vi "Optimal Frequency Bands Search.vi"() -> ()   [LabVIEW 2016]
uses:
  particle_swarm_opt/PSO_tParameters.ctl
  GA_core/GA_tParameters.ctl
  4. Accuracy Assessment for EEG Classification/_vlib/CU_ClassifierTypes.ctl
  <vilib>/Math Plots/2D Math Plots/2D Error Bar/2D Error Bar XCtrl/2D Error Bar.xctl
  4. Accuracy Assessment for EEG Classification/_vlib/CU_ClassifierQualityMeasure.ctl
  _vlib/OFBS_AlgorithmTypes.ctl
  _vlib/OFBS_metaParameters.ctl
  <vilib>/Math Plots/2D Math Plots/2D Error Bar/2D Error Bar Datatype/Public/Plot Helper (Fixed).vi
  4. Accuracy Assessment for EEG Classification/Classifier.lvlib
  <vilib>/Math Plots/2D Math Plots/2D Error Bar/2D Error Bar Datatype/2D Error Bar Datatype.lvclass
  <vilib>/Analysis/NI_AALBase.lvlib
  Optimal Frequency Bands Search.lvlib
  GA_core/GeneticAlgorithm.lvlib
  particle_swarm_opt/ParticleSwarm.lvlib
panel:
  in  "Stop Button":bool
  in  "Tab Control":T1(tab)
  in  "Algorithm Types":T2(tab)
  in  "GA parameters":T3={"Population size"=100, "Generations no."=20, "Significant digits"=5, "Crossover probabality"=0.85, "Mutation mode"=enum."one-point, fixed rate", "Use Gray code?"=TRUE, "Mutation rate"=0.05, "Min mutation rate"=0.0005, "Max mutation rate"=0.25, "Reproduction plan"=enum."Steady-state-replace-worst", "Elitism"=FALSE, "Fmax"=30} {"Max mutation rate" min=0.0 max=1.0; "Min mutation rate" min=0.0 max=1.0; "Mutation rate" min=0.0 max=1.0; "Crossover probabality" min=0.0 max=1.0; "Significant digits" min=1; "Generations no." min=1; "Population size" min=1}
  in  "PSO parameters":T4={"Swarm size"=100, "Generations no."=20, "Cognitive coeff a1"=2.05, "Social coeff a2"=2.05, "Min inertia weight"=0.4, "Max inertia weight "=0.9, "Fmax"=50} {"Generations no." min=1; "Swarm size" min=1}
  in  "Optimization Algorithm":T5 caption="Алгоритм поиска"
  in  "Number of Channels":i32=14 caption="Число каналов в записи ЭЭГ" min=1 max=128 step=1
  in  "ClassifierQualityMeasure":T6 caption="Критерий оценки точности классификации"
  in  "Use equal number of trials?":bool caption="Включить балансировку классов?"
  in  "Classifier Metaparameter":dbl=5.0 caption="Свободный параметр классификатора" min=0.0 max=100.0 step=0.1 format="%#_2g"
  in  "Iterations Num":i32=5
  in  "Training data paths":path[](array[path]) caption="Пути к файлам с обучающими данными"
  in  "Test data paths":path[](array[path]) caption="Пути к файлам с тестовыми данными"
  in  "True labels for Test data":path[](array[path]) caption="Пути к файлам с метками классов (для тестовых данных)"
  in  "ClassifierType":T7=enum."k NN Classifier" caption="Тип классификатора"
  in  "Start GA":bool
  out "Dataset Num":i32
  out "Total Progress":i32(slide) scale=0.0..25.0
  out "Solution":i32(listbox) caption="Оценки точности для решений, полученные после запусков поиска"
  out "Fitness Chart":cluster{i32[], dbl[]}[](graph) caption="Графики точности классификации"
  out "Accuracies":i32(listbox) caption="Оценки точности классификации на итерациях алгоритма поиска"
  out "Iteration":i32
  out "Results":string caption="Протокол выполнения программы"
  out "Accuracies out":dbl[][](array[numeric]) caption="Результаты"
  out "2D Error Bar":refnum<class "2D Plot Datatype.lvclass">[](xcontrol) caption="График средней точности классификации"
  # "This VI is a part of BCI Design library, http://www.ru-bci.org \nCopyright © 2020, Sotnikov Peter, All rights reserved. License: CC BY-NC 4.0"
  # "Параметры алгоритмов поиска"
  # "Число запусков ГА для каждого набора данных"
  # "Значение nu для SVM-классификатора (0,0 .. 1,0)\nЧисло соседей k для kNN-классификатора (1 .. 100)\nЧисло нейронов N скрытого слоя для многослойного персептрона (1 .. 100)"
  # "Размер популяции"
  # "Число поколений"
  # "Разрядность генома"
  # "Вероятность скрещивания"
  # "Тип мутаций"
  # "Использовать код Грея\nдля кодирования генома?"
  # "Вероятность мутации"
  # "Тип смены поколений"
  # "Fmax - верхняя граница частотного диапазона, \nFmin = 0"
  # "Размер роя"
  # "Число поколений"
  # "Коэффициент собственного лучшего значения"
  # "Коэффициент группового лучшего значения"
  # "Минимальное значение коэффициента инерции"
  # "Максимальное значение коэффициента инерции"
  # "Fmax - верхняя граница частотного диапазона, \nFmin = 0"
  # "Общее выполнение"
  # "Набор данных №"
  # "Запуск ГА №"
  # "Среднее \nпо наборам"
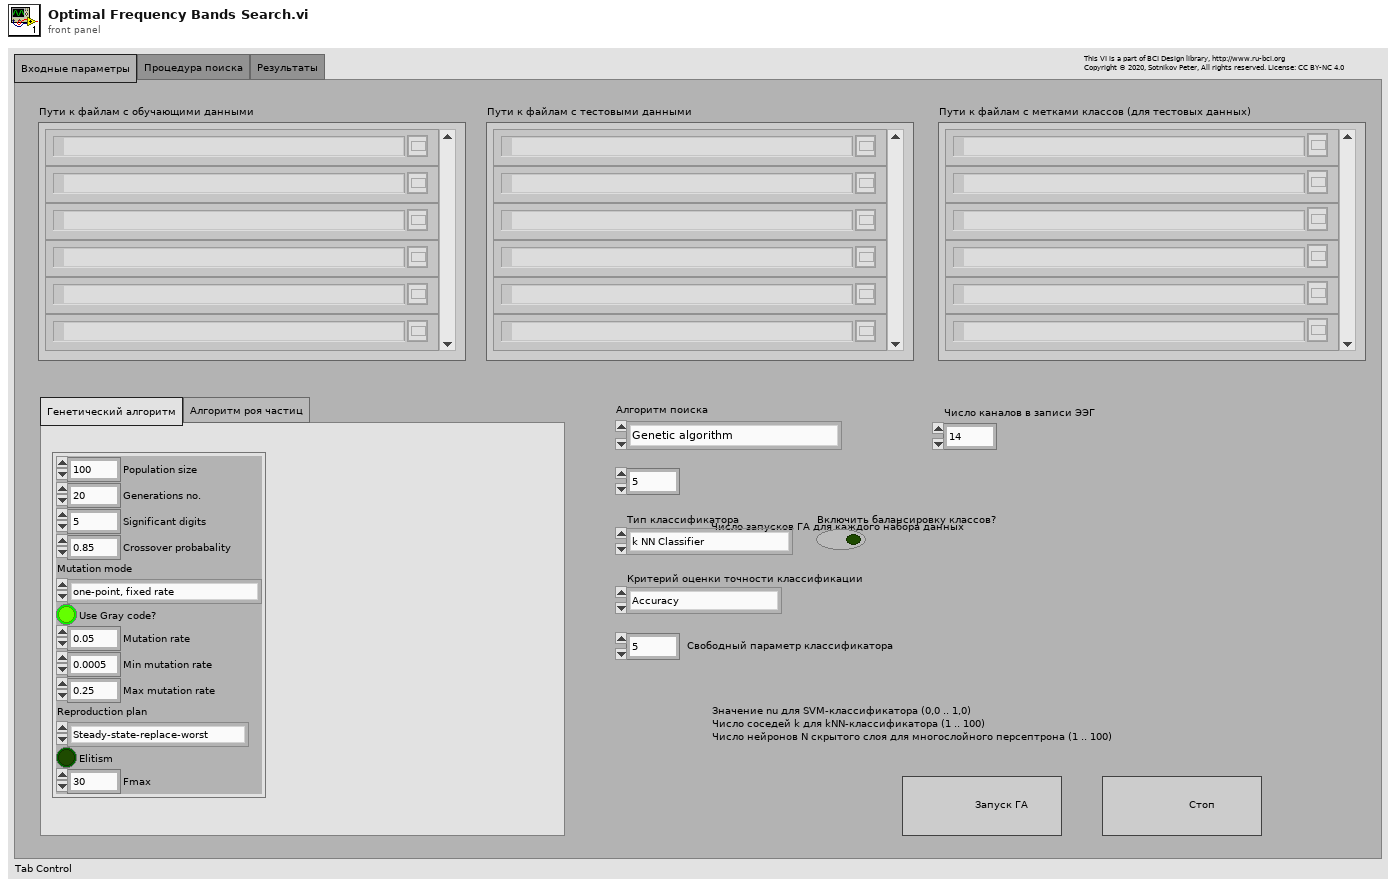
[diagram p1: front panel]
types:
  T1 = enum32{"Входные параметры", "Процедура поиска", "Результаты"}
  T2 = enum32{"Генетический алгоритм", "Алгоритм роя частиц"}
  T3 = typedef "Optimal Frequency Bands Search.lvlib/GeneticAlgorithm.lvlib/GA_tParameters.ctl" = cluster{"Population size":i32, "Generations no.":i32, "Significant digits":i32, "Crossover probabality":dbl, "Mutation mode":enum16{"one-point, fixed rate", "one-point, fitness-adjustable rate", "one-point, distance-adjustable rate"}, "Use Gray code?":bool, "Mutation rate":dbl, "Min mutation rate":dbl, "Max mutation rate":dbl, "Reproduction plan":enum16{"Full generational replacement", "Steady-state-replace-random", "Steady-state-replace-worst"}, "Elitism":bool, "Fmax":i32}
  T4 = typedef "Optimal Frequency Bands Search.lvlib/ParticleSwarm.lvlib/PSO_tParameters.ctl" = cluster{"Swarm size":i32, "Generations no.":i32, "Cognitive coeff a1":dbl, "Social coeff a2":dbl, "Min inertia weight":dbl, "Max inertia weight ":dbl, "Fmax":i32}
  T5 = typedef "Optimal Frequency Bands Search.lvlib/OFBS_AlgorithmTypes.ctl" = enum16{"Genetic algorithm", "Particle swarm optimization"}
  T6 = typedef "Classifier.lvlib/CU_ClassifierQualityMeasure.ctl" = enum16{"Accuracy", "Cohen's kappa"}
  T7 = typedef "Classifier.lvlib/CU_ClassifierTypes.ctl" = enum16{"Multilayer perceptron", "k NN Classifier", "SVM Committee", "Mahalanobis distance", "SVM Classifier"}
  T8 = typedef "Optimal Frequency Bands Search.lvlib/OFBS_metaParameters.ctl" = cluster{"Training Data Path":path, "Test Data Path":path, "True Labels for Test Trials":path, "Optimization Algorithm":T5, "ClassifierType":T7, "GA Parameters":T3, "PSO Parameters":T4, "Number of Channels":i32, "Use equal number of trials?":bool, "Classifier Metaparameter":dbl, "ClassifierQualityMeasure":T6}
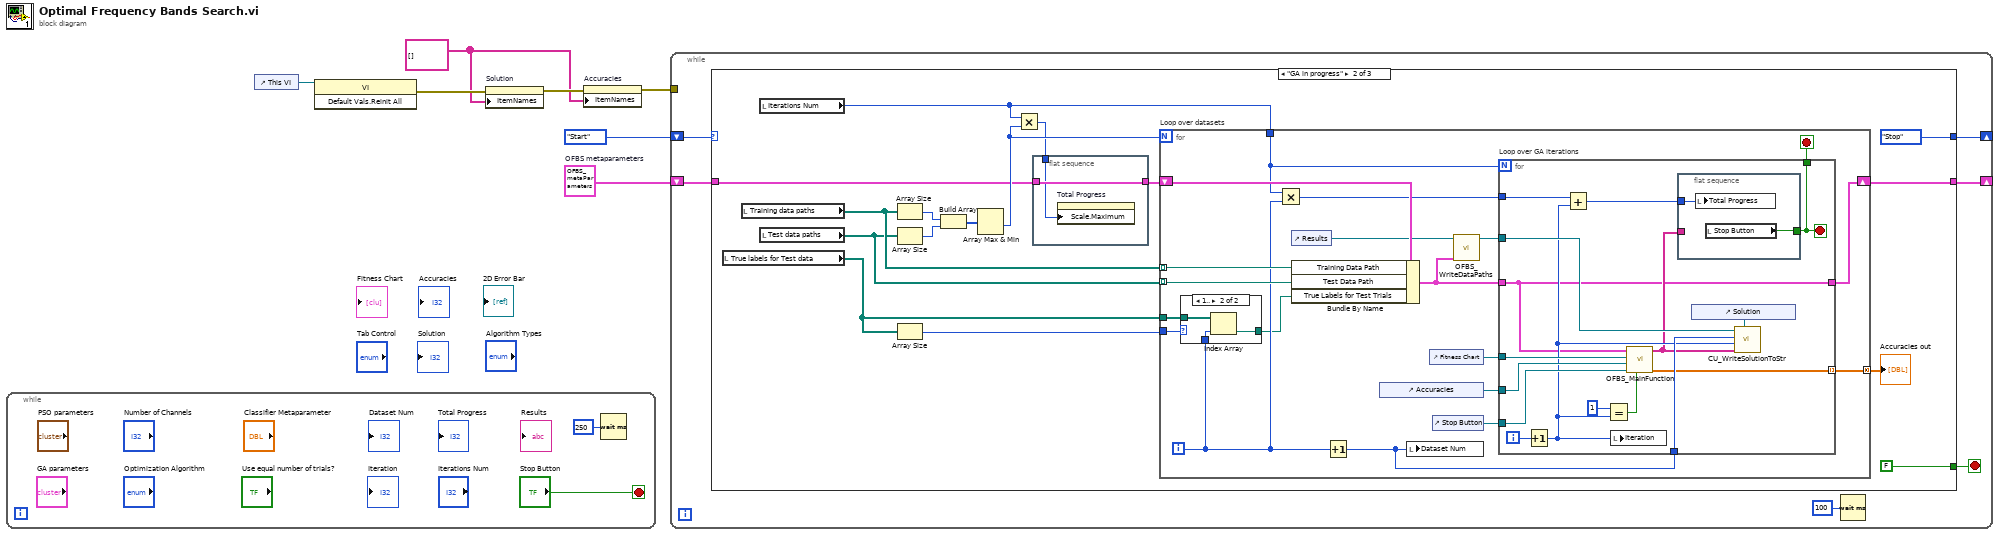
[diagram p0: block diagram]
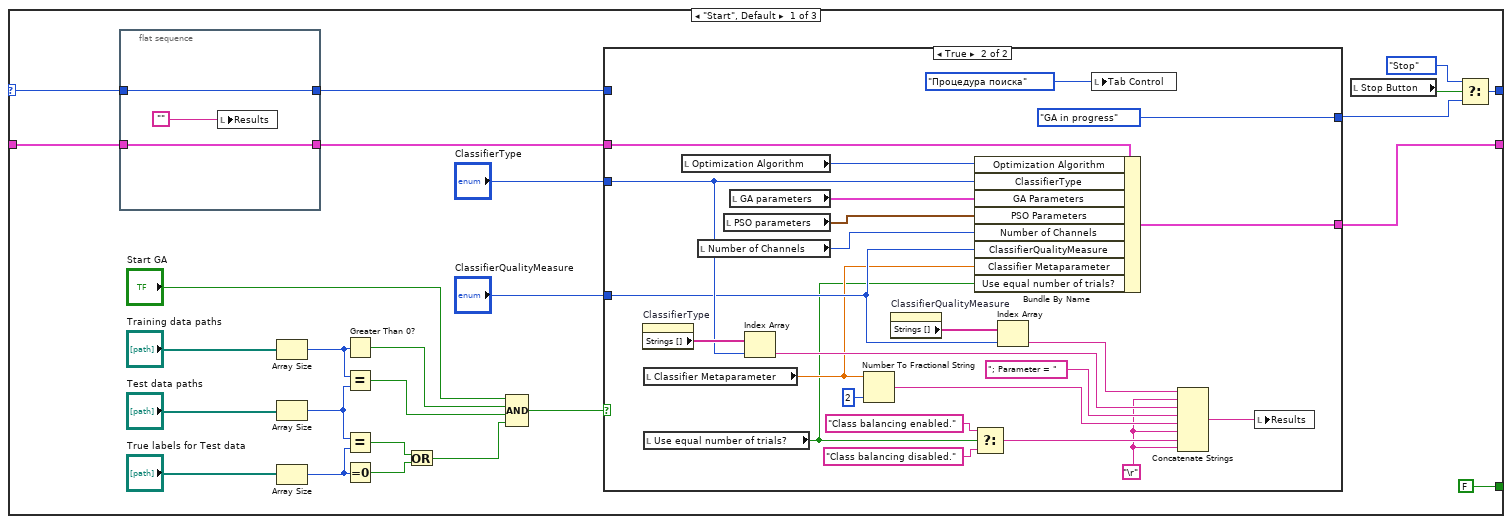
[diagram p2: hidden frame]
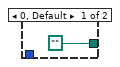
[diagram p4: hidden frame]
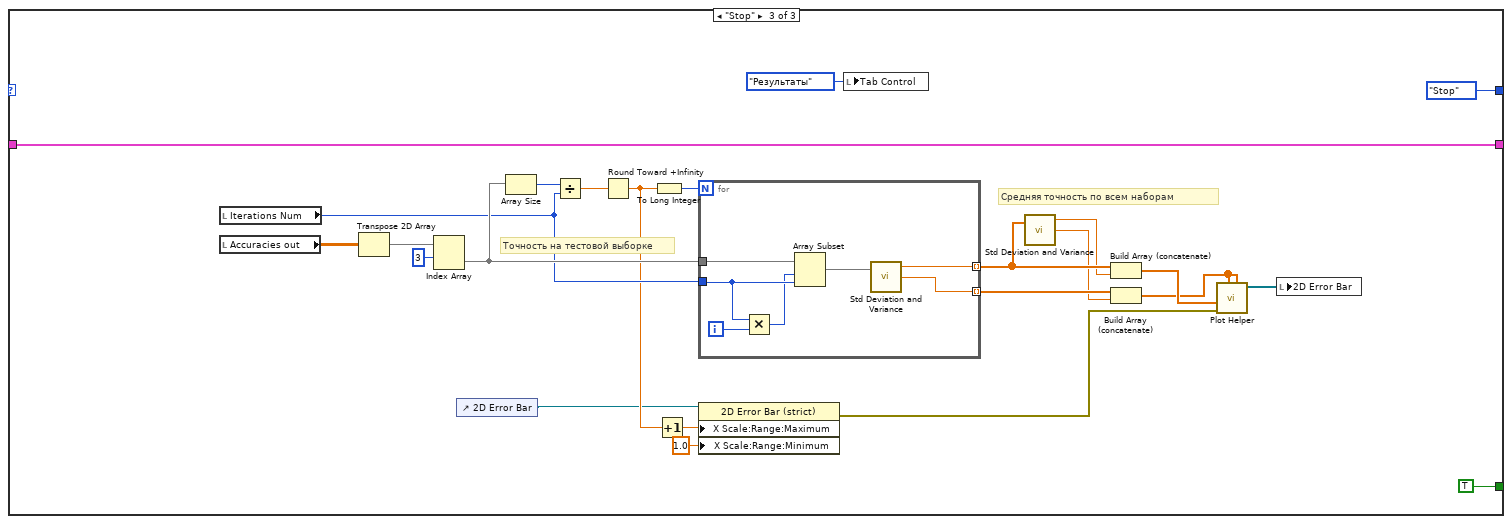
[diagram p5: hidden frame]
diagram:
  w1 = string[][] [] ("Item Names")
  w6 = T8 {"Training Data Path"=path "", "Test Data Path"=path "", "True Labels for Test Trials"=path "", "Optimization Algorithm"=enum."Genetic algorithm", "ClassifierType"=enum."Multilayer perceptron", "GA Parameters"={"Population size"=100, "Generations no."=500, "Significant digits"=4, "Crossover probabality"=0.85, "Mutation mode"=enum."one-point, fixed rate", "Use Gray code?"=FALSE, "Mutation rate"=0.05, "Min mutation rate"=0.0005, "Max mutation rate"=0.25, "Reproduction plan"=enum."Steady-state-replace-worst", "Elitism"=FALSE, "Fmax"=1}, "PSO Parameters"={"Swarm size"=50, "Generations no."=10, "Cognitive coeff a1"=2.05, "Social coeff a2"=2.05, "Min inertia weight"=0.4, "Max inertia weight "=0.9, "Fmax"=0}, "Number of Channels"=5, "Use equal number of trials?"=FALSE, "Classifier Metaparameter"=0.0, "ClassifierQualityMeasure"=enum."Accuracy"}  # OFBS metaparameters
  n1 = while {
    stop <- "Stop Button" stop-if-true
    n2 = Wait (ms)(milliseconds to wait=u32 250) -> ()  [unwired: 1 out]
  }
  n3 = control-ref of="This VI"() -> (w5:refnum<vi>)
  n4 = invoke class="VI" method="Default Vals.Reinit All"(reference=w5) -> (error out=w4:errorcluster)  [unwired: 2 in, 2 out]
  n5 = property on="Solution" class="MCListbox (strict)"(error in=w4, "ItemNames"=w1) -> (error out=w3:errorcluster)  [unwired: 1 in, 1 out]
  n6 = property on="Accuracies" class="MCListbox (strict)"(error in=w3, "ItemNames"=w1) -> (error out=w2:errorcluster)  [unwired: 1 in, 1 out]
  n7 = while {
    shift-right: [w12] -> _
    shift-left: w6 -> [w14]
    shift-right: [w13] -> _
    shift-left: enum16{"Start", "GA in progress", "Stop"}."Start" -> [w15]
    tunnel: w2 -> [_]
    stop <- w10 stop-if-true
    n8 = case shown="\"GA in progress\"" w15 {
      selector: w15 -> [w27 _ _]
      tunnel: w14 -> [w25 w71 w150]
      tunnel: [w31 enum16{"Start", "GA in progress", "Stop"}."Stop" ("t") enum16{"Start", "GA in progress", "Stop"}."Stop"] -> w13
      tunnel: [w33 w77 w150] -> w12
      tunnel: [FALSE FALSE TRUE] -> w10
      frame "Start", Default {
        n9 = flat-sequence {
          tunnel: w27 -> [w43]
          tunnel: [w43] -> w26
          tunnel: w25 -> [w42]
          tunnel: [w42] -> w24
          frame #0 {
            n10 = local write "Results"("") -> ()
          }
        }
        n11 = Array Size(array="Training data paths") -> (size(s)=w23:i32)
        n12 = Array Size(array="Test data paths") -> (size(s)=w40:i32)
        n13 = Array Size(array="True labels for Test data") -> (size(s)=w22:i32)
        n14 = Greater Than 0?(x=w23) -> (x > 0?=w17:bool)
        n15 = Equal?(x=w23, y=w40) -> (x = y?=w18:bool)
        n16 = Equal?(x=w40, y=w22) -> (x = y?=w21:bool)
        n17 = Equal To 0?(x=w22) -> (x = 0?=w20:bool)
        n18 = Or(x=w21, y=w20) -> (x .or. y?=w19:bool)
        n19 = Compound Arithmetic op=AND("Start GA", w17, w18, w19) -> (w39:bool)
        n20 = case shown="True" w39 {
          tunnel: w24 -> [w45 w69]
          tunnel: "ClassifierType" -> [_ w65]
          tunnel: w26 -> [w44 _]
          tunnel: [w44 enum16{"Start", "GA in progress", "Stop"}."GA in progress"] -> w29
          tunnel: [w45 w67] -> w33
          tunnel: "ClassifierQualityMeasure" -> [_ w48]
          frame False {
          }
          frame True {
            w56 = "\r"
            n21 = property on="ClassifierType" class="Enum (strict)"() -> ("Strings []"=w66:string[])  [unwired: 2 in, 2 out]
            n22 = local read "Classifier Metaparameter"() -> (w47:dbl)
            n23 = local read "Use equal number of trials?"() -> (w46:bool)
            n24 = local read "Optimization Algorithm"() -> (w52:T5)
            n25 = local read "Number of Channels"() -> (w49:i32)
            n26 = local read "PSO parameters"() -> (w50:T4)
            n27 = local read "GA parameters"() -> (w51:T3)
            n28 = Index Array(array=w66, index=w65) -> (element=w60:string)
            n29 = Number To Fractional String(number=w47, precision (6)=i16 2) -> (F-format string=w58:string)  [unwired: 2 in]
            n30 = property on="ClassifierQualityMeasure" class="Enum (strict)"() -> ("Strings []"=w55:string[])  [unwired: 2 in, 2 out]
            n31 = Bundle By Name(cluster=w69, "Optimization Algorithm"=w52, "ClassifierType"=w65, "GA Parameters"=w51, "PSO Parameters"=w50, "Number of Channels"=w49, "ClassifierQualityMeasure"=w48, "Classifier Metaparameter"=w47, "Use equal number of trials?"=w46) -> (w67:T8)
            n32 = Select(t="Class balancing enabled.", s=w46, f="Class balancing disabled.") -> (s? t:f=w57:string)
            n33 = Index Array(array=w55, index=w48) -> (element=w54:string)
            n34 = local write "Tab Control"(T1."Процедура поиска" ("Tab Control")) -> ()
            n35 = Concatenate Strings(w54, w56, w60, "; Parameter = ", w58, w56, w57, w56) -> (w64:string)
            n36 = local write "Results"(w64) -> ()
          }
        }
        n37 = local read "Stop Button"() -> (w30:bool)
        n38 = Select(t=enum16{"Start", "GA in progress", "Stop"}."Stop", s=w30, f=w29) -> (s? t:f=w31:enum16{"Start", "GA in progress", "Stop"})
      }
      frame "GA in progress" {
        n39 = local read "True labels for Test data"() -> (w79:path[])
        n40 = local read "Training data paths"() -> (w81:path[])
        n41 = local read "Iterations Num"() -> (w75:i32)
        n42 = local read "Test data paths"() -> (w80:path[])
        n43 = Array Size(array=w81) -> (size(s)=w84:i32)
        n44 = Array Size(array=w80) -> (size(s)=w83:i32)
        n45 = Array Size(array=w79) -> (size(s)=w73:i32)
        n46 = Build Array(w84, w83) -> (w82:i32[])
        n47 = Array Max & Min(array=w82) -> (min value=w74:i32)  [unwired: 3 out]
        n48 = Multiply(x=w75, y=w74) -> (x*y=w70:i32)
        n49 = flat-sequence {
          tunnel: [w87] -> w72
          tunnel: w71 -> [w87]
          tunnel: w70 -> [w86]
          frame #0 {
            n50 = property on="Total Progress" class="Slide (strict)"("Scale.Maximum"=w86) -> ()  [unwired: 2 in, 2 out]
          }
        }
        n51 = for "Loop over datasets" {
          N: w74 -> [_]
          tunnel: w81 -> [w105] mode=indexing
          tunnel: w80 -> [w104] mode=indexing
          tunnel: w79 -> [w90]
          shift-right: [w100] -> w77
          shift-left: w72 -> [w106]
          tunnel: [w98] -> w76 mode=concatenating
          tunnel: w75 -> [w97]
          tunnel: w73 -> [w91]
          i -> [w92]
          stop <- w99 stop-if-true
          n52 = case shown="1.." w91 {
            tunnel: w90 -> [_ w110]
            tunnel: w92 -> [_ w109]
            tunnel: [path "" w108] -> w89
            frame 0, Default {
            }
            frame 1.. {
              n53 = Index Array(array=w110, index=w109) -> (element=w108:path)
            }
          }
          n54 = Multiply(x=w97, y=w92) -> (x*y=w96:i32)
          n55 = control-ref of="Results"() -> (w95:refnum<vi>)
          n56 = Bundle By Name(cluster=w106, "Training Data Path"=w105, "Test Data Path"=w104, "True Labels for Test Trials"=w89) -> (w88:T8)
          n57 = Increment(x=w92) -> (x+1=w93:i32)
          n58 = control-ref of="Accuracies"() -> (w102:refnum<vi>)
          n59 = local write "Dataset Num"(w93) -> ()
          n60 = control-ref of="Fitness Chart"() -> (w103:refnum<vi>)
          n61 = control-ref of="Stop Button"() -> (w101:refnum<vi>)
          n62 = call "OFBS_WriteDataPaths.vi"("OFBS metaparameters in"=w88, "String Ref in"=w95) -> ("String Ref out"=w94:refnum<vi>)  [unwired: 7 in, 2 out]
          n63 = for "Loop over GA iterations" {
            N: w97 -> [_]
            tunnel: w88 -> [w113]
            tunnel: w103 -> [w126]
            tunnel: w102 -> [w125]
            tunnel: w101 -> [w124]
            tunnel: [w112] -> w98 mode=indexing
            tunnel: [w113] -> w100
            tunnel: [w123] -> w99
            tunnel: w96 -> [w122]
            tunnel: w94 -> [w119]
            tunnel: w93 -> [w117]
            i -> [w121]
            stop <- w123 stop-if-true
            n64 = Increment(x=w121) -> (x+1=w116:i32)
            n65 = Add(x=w122, y=w116) -> (x+y=w120:i32)
            n66 = Equal?(x=1, y=w116) -> (x = y?=w111:bool)
            n67 = local write "Iteration"(w116) -> ()
            n68 = call "OFBS_MainFunction.vi"("ReInitialize?"=w111, "Stop ButtonRef in"=w124, "Results ListBox Ref"=w125, "Fitness Chart Ref in"=w126, "OFBS metaparameters in"=w113) -> ("Results dbl"=w112:dbl[], "Results str"=w114:string[])  [unwired: 5 in]
            n69 = flat-sequence {
              tunnel: [w128] -> w123
              tunnel: w120 -> [w127]
              tunnel: w114 -> [_]
              frame #0 {
                n70 = local write "Total Progress"(w127) -> ()
                n71 = local read "Stop Button"() -> (w128:bool)
              }
            }
            n72 = control-ref of="Solution"() -> (w118:refnum<vi>)
            n73 = call "CU_WriteSolutionToStr.vi"("ListBox Ref in"=w118, "Solution in"=w114, "Iteration Num"=w116, "Dataset Num"=w117, "String Ref in"=w119) -> ()  [unwired: 5 in, 2 out]
          }
        }
        "Accuracies out" <- w76
      }
      frame "Stop" {
        # "Средняя точность по всем наборам"
        # "Точность на тестовой выборке"
        n74 = local read "Iterations Num"() -> (w143:i32)
        n75 = local read "Accuracies out"() -> (w149:dbl[][])
        n76 = Transpose 2D Array(2D array=w149) -> (transposed array=w148:dbl[][])
        n77 = Index Array(array=w148, index (row)=3) -> (element=w144:dbl[])  [unwired: 1 in]
        n78 = control-ref of="2D Error Bar"() -> (w130:refnum<vi>)
        n79 = Array Size(array=w144) -> (size(s)=w146:i32)
        n80 = Divide(x=w146, y=w143) -> (x/y=w145:dbl)
        n81 = Round Toward +Infinity(x=w145) -> (ceil(x): smallest int >= x=w132:dbl)
        n82 = To Long Integer(number=w132) -> (32bit integer=w133:i32)
        n83 = Increment(x=w132) -> (x+1=w135:dbl)
        n84 = for {
          N: w133 -> [_]
          tunnel: w144 -> [w159]
          tunnel: w143 -> [w158]
          tunnel: [w155] -> w142 mode=indexing
          tunnel: [w154] -> w140 mode=indexing
          i -> [w153]
          n85 = Multiply(x=w158, y=w153) -> (x*y=w157:i32)
          n86 = Array Subset(array=w159, index=w157, length=w158) -> (w156:dbl[])
          n87 = call <vilib>:"Std Deviation and Variance.vi"("X"=w156) -> ("mean"=w155:dbl, "standard deviation"=w154:dbl)  [unwired: 1 in, 1 out]
        }
        n88 = property class="2D Error Bar (strict)"(reference=w130, "X Scale:Range:Maximum"=w135, "X Scale:Range:Minimum"=1.0) -> (error out=w134:errorcluster)  [unwired: 1 in, 1 out]
        n89 = local write "Tab Control"(T1."Результаты" ("Tab Control")) -> ()
        n90 = call <vilib>:"Std Deviation and Variance.vi"("X"=w142) -> ("mean"=w141:dbl, "standard deviation"=w139:dbl)  [unwired: 1 in, 1 out]
        n91 = Build Array (concatenate)(w142, w141) -> (w138:dbl[])
        n92 = Build Array (concatenate)(w140, w139) -> (w137:dbl[])
        n93 = call-poly <vilib>:"Plot Helper.vi"("error b vector"=w137, "error a vector"=w137, "error in (no error)"=w134, "y vector"=w138) -> ("2D Plot Class Obj Array out"=w136:refnum<class "2D Plot Datatype.lvclass">[])  [unwired: 2 in, 5 out]
        n94 = local write "2D Error Bar"(w136) -> ()
      }
    }
    n95 = Wait (ms)(milliseconds to wait=u32 100) -> ()  [unwired: 1 out]
  }
